vi "RFIDGetTagPresent.vi"(0 "error in (no error)":errorcluster, 3 "Device In":u64) -> (7 "error out":errorcluster, 9 "Tag State":bool caption="Tag Present", 10 "Device Out":u64)   [LabVIEW 2012, in "Phidget RFID.lvlib"]
doc: "${TagPresent:Header}"
uses:
  <instrlib>/Phidgets/Phidget RFID/Phidget RFID.lvlib
  <instrlib>/Phidgets/Phidget Common/Phidget Common.lvlib
  phidget22.dll
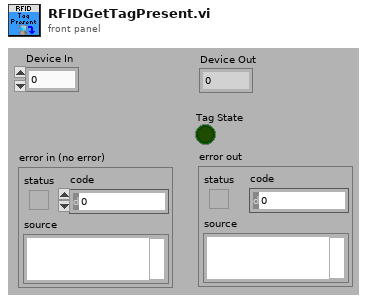
[diagram p1: front panel]
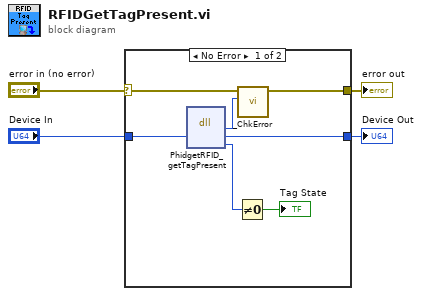
[diagram p0: block diagram]
diagram:
  n1 = case shown="No Error" "error in (no error)" {
    selector: "error in (no error)" -> [w8 w13]
    tunnel: [w7 w13] -> w3
    tunnel: "Device In" -> [w11 w12]
    tunnel: [w10 w12] -> w1
    frame No Error {
      n2 = dll-call lib="phidget22.*" fn="PhidgetRFID_getTagPresent"("phid"=w11) -> ("return type"=w9:i32, "phid"=w10:u64, "EngagedState_out"=w6:i32)  [unwired: 4 in, 2 out]
      n3 = Not Equal To 0?(x=w6) -> (x != 0?=→"Tag State":bool)
      n4 = call <instrlib>:"_ChkError.vi"("Return Code"=w9, "error in (no error)"=w8) -> ("error out"=w7:errorcluster)  [unwired: 9 in]
    }
    frame Error {
    }
  }
  "error out" <- w3
  "Device Out" <- w1
